vi "Progressbar.vi"() -> ()   [LabVIEW 2015]
panel:
  out "Progress":u8(slide) max=100 scale=0.0..100.0
  # "% Complete"
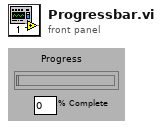
[diagram p1: front panel]
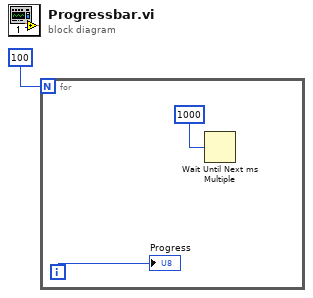
[diagram p0: block diagram]
diagram:
  n1 = for {
    N: 100 -> [_]
    i -> [w3]
    n2 = Wait Until Next ms Multiple(millisecond multiple=1000) -> ()  [unwired: 1 out]
    "Progress" <- w3
  }
